vi "Index_Array_2D_SubArray.vi"(9 "Index Array 2D":i8[][](array[numeric])=[[0, 4, -3], [1, 5, -4], [2, -1, -5], [3, -2, 100]], 10 "Indexs IA":T1={"Rows"=-1, "Columns"=-1} {"Columns" min=-1; "Rows" min=-1}) -> (2 "Index SubArray":i8[](array[numeric]))   [LabVIEW 2018]
uses:
  Controls/Rows_Columns.ctl
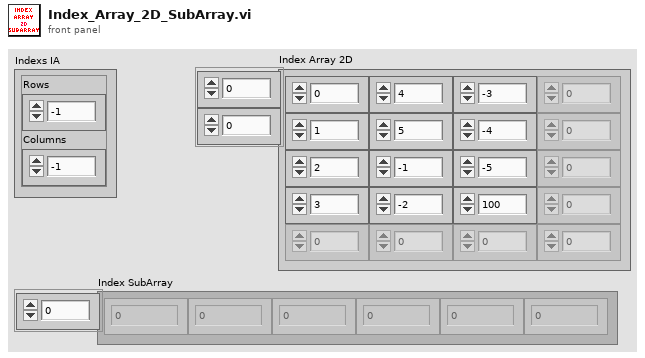
[diagram p1: front panel]
types:
  T1 = typedef "Rows_Columns.ctl" = cluster{"Rows":i32, "Columns":i32}
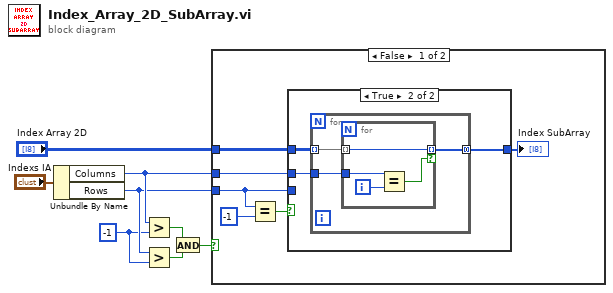
[diagram p0: block diagram]
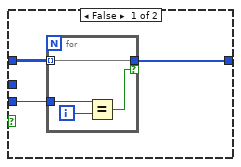
[diagram p2: hidden frame]
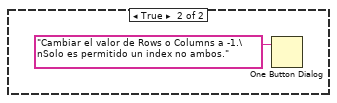
[diagram p3: hidden frame]
diagram:
  w1 = -1 ("y")
  n1 = Unbundle By Name("Indexs IA") -> ("Columns"=w3:i32, "Rows"=w2:i32)
  n2 = Greater?(x=w3, y=w1) -> (0:w5:bool)
  n3 = Greater?(x=w2, y=w1) -> (0:w4:bool)
  n4 = And(x=w5, y=w4) -> (x .and. y?=w6:bool)
  n5 = case shown="False" w6 {
    tunnel: "Index Array 2D" -> [w14 _]
    tunnel: w2 -> [w11 _]
    tunnel: w3 -> [w10 _]
    frame False {
      n6 = Equal?(x=w11, y=-1) -> (x = y?=w12:bool)
      n7 = case shown="True" w12 {
        tunnel: w14 -> [w17 w24]
        tunnel: [w15 w23] -> w9
        tunnel: w11 -> [w16 _]
        tunnel: w10 -> [_ w22]
        frame False {
          n8 = for {
            tunnel: w17 -> [w18] mode=indexing
            tunnel: [w18] -> w15 if=w21
            tunnel: w16 -> [w20]
            i -> [w19]
            n9 = Equal?(x=w20, y=w19) -> (x = y?=w21:bool)
          }
        }
        frame True {
          n10 = for {
            tunnel: w24 -> [w27] mode=indexing
            tunnel: [w26] -> w23 mode=concatenating
            tunnel: w22 -> [w25]
            n11 = for {
              tunnel: w27 -> [w31] mode=indexing
              tunnel: [w31] -> w26 mode=indexing if=w30
              tunnel: w25 -> [w28]
              i -> [w29]
              n12 = Equal?(x=w28, y=w29) -> (x = y?=w30:bool)
            }
          }
        }
      }
      "Index SubArray" <- w9
    }
    frame True {
      n13 = One Button Dialog(message="Cambiar el valor de Rows o Columns a -1.\nSolo es permitido un index no ambos.") -> ()  [unwired: 1 in, 1 out]
    }
  }
